vi "HV_Test.vi"(8 "Error In":errorcluster, 10 "PORT":string, 11 "Limit":string) -> (0 "error out":errorcluster, 2 "Result":bool, 3 "Data":string)   [LabVIEW 2013]
uses:
  MainProgram/Control/Buffer.vi
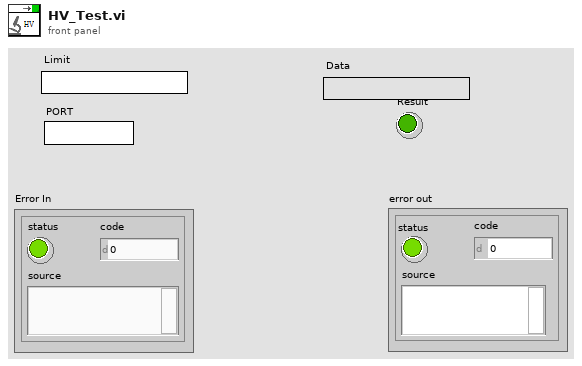
[diagram p1: front panel]
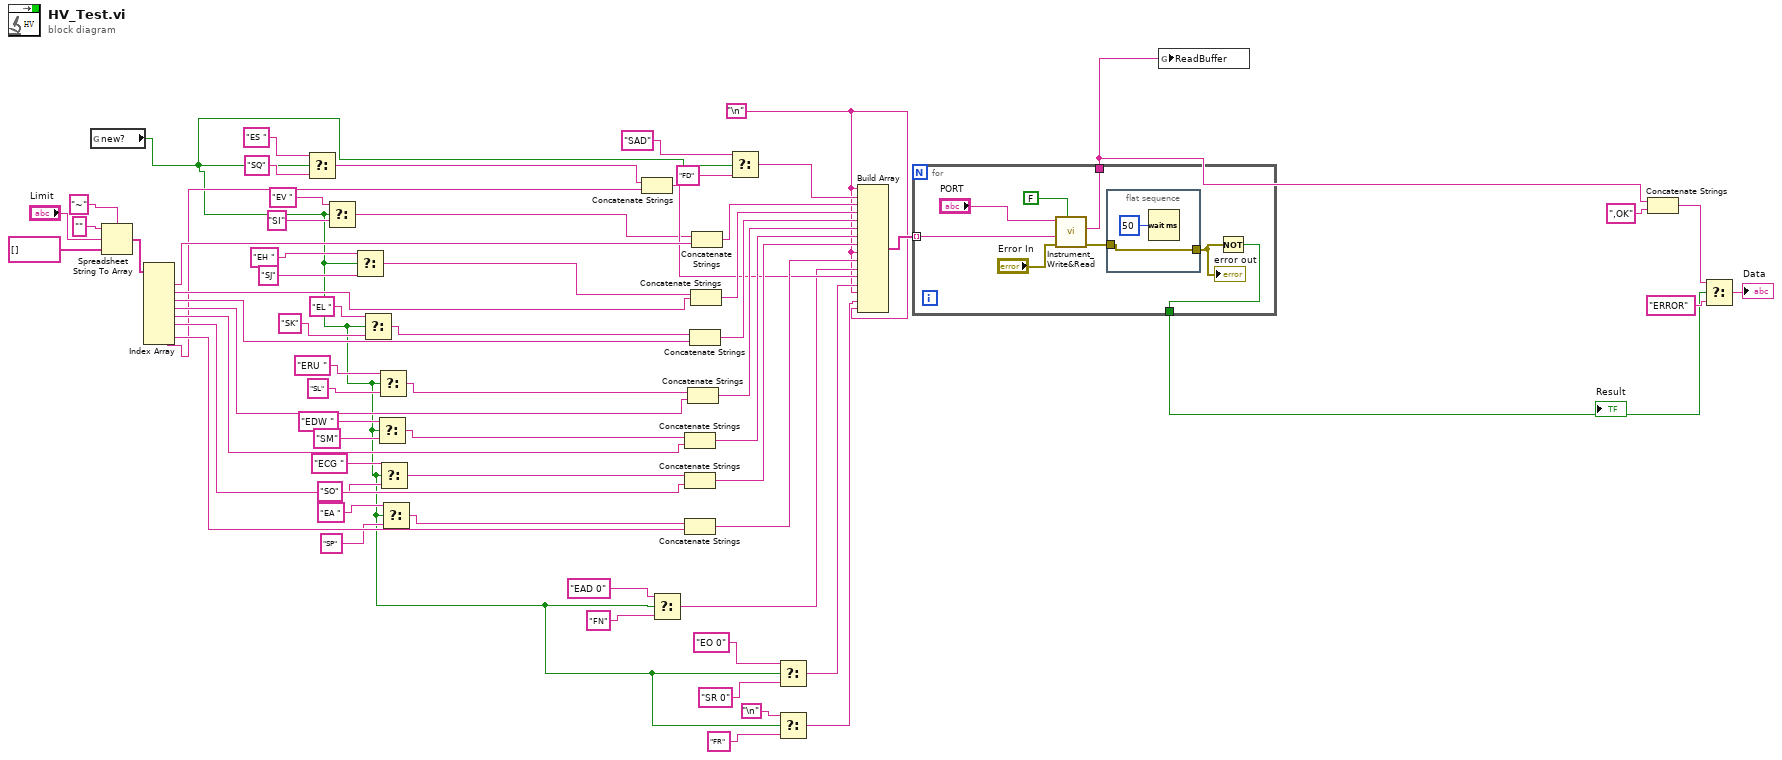
[diagram p0: block diagram]
diagram:
  w2 = "\n"
  n1 = global read "Buffer.vi" "new?"() -> (w5:bool)
  n2 = Spreadsheet String To Array(delimiter (Tab)="~", format string="", spreadsheet string="Limit", array type (2D Dbl)=string[] []) -> (array=w60:string[])
  n3 = Index Array(array=w60) -> (element #1=w54:string, element #2=w51:string, element #3=w50:string, element #4=w47:string, element #5=w46:string, element #6=w43:string, element #7=w41:string, element #8=w39:string)  [unwired: 8 in]
  n4 = Select(t="ES " ("element"), s=w5, f="SQ" ("element")) -> (s? t:f=w37:string)
  n5 = Select(t="EV " ("string"), s=w5, f="SI" ("string")) -> (s? t:f=w34:string)
  n6 = Select(t="EH " ("string"), s=w5, f="SJ" ("string")) -> (s? t:f=w31:string)
  n7 = Select(t="EL " ("string"), s=w5, f="SK" ("string")) -> (s? t:f=w28:string)
  n8 = Select(t="EDW " ("string"), s=w5, f="SM" ("string")) -> (s? t:f=w22:string)
  n9 = Select(t="ERU " ("string"), s=w5, f="SL" ("string")) -> (s? t:f=w25:string)
  n10 = Select(t="ECG " ("string"), s=w5, f="SO" ("string")) -> (s? t:f=w19:string)
  n11 = Select(t="EA " ("string"), s=w5, f="SP" ("string")) -> (s? t:f=w16:string)
  n12 = Concatenate Strings(w37, w39) -> (w40:string)
  n13 = Select(t="EAD 0" ("element"), s=w5, f="FN" ("element")) -> (s? t:f=w10:string)
  n14 = Concatenate Strings(w22, w46) -> (w45:string)
  n15 = Concatenate Strings(w19, w43) -> (w44:string)
  n16 = Concatenate Strings(w16, w41) -> (w42:string)
  n17 = Concatenate Strings(w25, w47) -> (w48:string)
  n18 = Concatenate Strings(w28, w50) -> (w49:string)
  n19 = Concatenate Strings(w31, w51) -> (w52:string)
  n20 = Concatenate Strings(w34, w54) -> (w53:string)
  n21 = Select(t="SAD" ("format string"), s=w5, f="FD" ("format string")) -> (s? t:f=w13:string)
  n22 = Select(t="EO 0" ("element"), s=w5, f="SR 0" ("element")) -> (s? t:f=w6:string)
  n23 = Select(t="\n", s=w5, f="FR" ("element")) -> (s? t:f=w3:string)
  n24 = Build Array(w2, w13, w53, w52, w49, w48, w45, w44, w2, w42, w10, w40, w6, w2, w3, w2) -> (w55:string[])
  n25 = for {
    tunnel: [w74] -> w64
    tunnel: [w70] -> w56
    tunnel: w55 -> [w69] mode=indexing
    n26 = call "Instrument_Write&Read.vi"("Read?"=FALSE, "Error In"="Error In", "CMD"=w69, "PORT"="PORT") -> ("Error Out"=w67:errorcluster, "read buffer"=w70:string)  [unwired: 6 in]
    n27 = flat-sequence {
      tunnel: [w76] -> w68
      tunnel: w67 -> [w76]
      frame #0 {
        n28 = Wait (ms)(milliseconds to wait=u32 50) -> ()  [unwired: 1 out]
      }
    }
    n29 = Not(x=w68) -> (.not. x?=w74:bool)
    "error out" <- w68
  }
  "Result" <- w64
  n30 = global write "Buffer.vi" "ReadBuffer"(w56) -> ()
  n31 = Concatenate Strings(w56, ",OK") -> (w57:string)
  n32 = Select(t=w57, s=w64, f="ERROR") -> (s? t:f=→"Data":string)
